vi "Service Mode Test Data.vi"(5 "High\\Low End":enum16{"HE", "LE"}(ring), 9 "Switch":T1=enum."Test 1 - Fault Codes") -> (8 "Switch Message":string)   [LabVIEW 2016, in "TL27.lvlib"]
uses:
  Projects/TL27.lvlib
  type defs/Service mode Tests.ctl
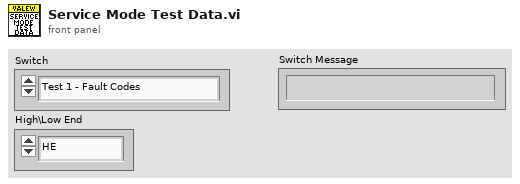
[diagram p1: front panel]
types:
  T1 = typedef "TL27.lvlib/Service mode Tests.ctl" = enum16{"Test 0 - All LEDs on", "Test 1 - Fault Codes", "Test 2 - Personality ID", "Test 3 - UI Software Ver(Crit)", "Test 4 - UI Software Ver(Non-crit)", "Test 5 - XML Ver (Non-Crit) ", "Test 6 - Hot Water Valve", "Test 7 - Cold Water Valve", "Test 8 - Fabric Softener Disp", "Test 9 - Spray Rinse Valve Check", "Test 10 - Pressure Sensor", "Test 11 - Recirc Pump", "Test 12 - Drain Pump", "Test 13 - Lid Switch", "Test 14 - Spin", "Test 15 - Agitate", "Test 16 - Clear all Fcodes", "Test 17 - Change Personality", "Test 18 - Analog Knob", "Test 19 - Bulk Dispense"}
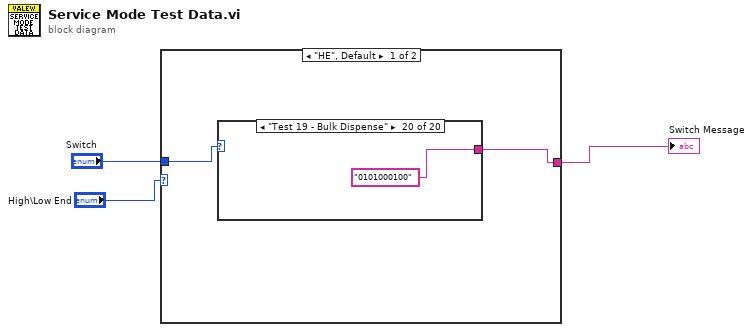
[diagram p0: block diagram]
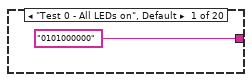
[diagram p2: hidden frame]
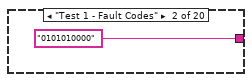
[diagram p3: hidden frame]
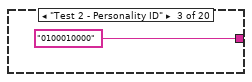
[diagram p4: hidden frame]
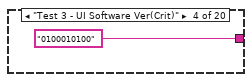
[diagram p5: hidden frame]
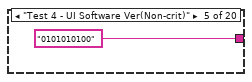
[diagram p6: hidden frame]
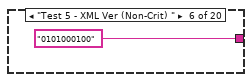
[diagram p7: hidden frame]
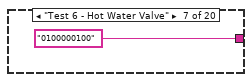
[diagram p8: hidden frame]
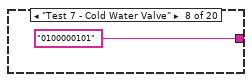
[diagram p9: hidden frame]
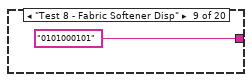
[diagram p10: hidden frame]
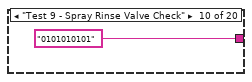
[diagram p11: hidden frame]
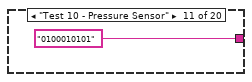
[diagram p12: hidden frame]
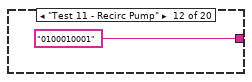
[diagram p13: hidden frame]
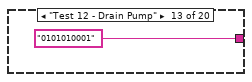
[diagram p14: hidden frame]
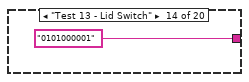
[diagram p15: hidden frame]
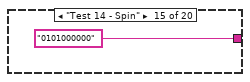
[diagram p16: hidden frame]
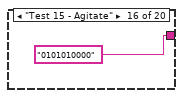
[diagram p17: hidden frame]
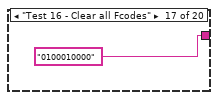
[diagram p18: hidden frame]
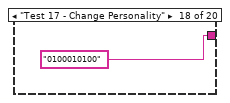
[diagram p19: hidden frame]
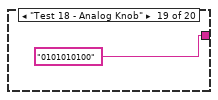
[diagram p20: hidden frame]
diagram:
  n1 = case shown="\"HE\", Default" "High\\Low End" {
    tunnel: [w4 w26] -> w3
    tunnel: "Switch" -> [w5 w27]
    frame "HE", Default {
      n2 = case shown="\"Test 19 - Bulk Dispense\"" w5 {
        tunnel: ["0101000000" ("Message") "0101010000" ("Message") "0100010000" ("Message") "0100010100" ("Message") "0101010100" ("Message") "0101000100" ("Message") "0100000100" ("Message") "0100000101" ("Message") "0101000101" ("Message") "0101010101" ("Message") "0100010101" ("Message") "0100010001" ("Message") "0101010001" ("Message") "0101000001" ("Message") "0101000000" ("Message") "0101010000" ("Message") "0100010000" ("Message") "0100010100" ("Message") "0101010100" ("Message") "0101000100" ("Message")] -> w4
        frame "Test 0 - All LEDs on", Default {
        }
        frame "Test 1 - Fault Codes" {
        }
        frame "Test 2 - Personality ID" {
        }
        frame "Test 3 - UI Software Ver(Crit)" {
        }
        frame "Test 4 - UI Software Ver(Non-crit)" {
        }
        frame "Test 5 - XML Ver (Non-Crit) " {
        }
        frame "Test 6 - Hot Water Valve" {
        }
        frame "Test 7 - Cold Water Valve" {
        }
        frame "Test 8 - Fabric Softener Disp" {
        }
        frame "Test 9 - Spray Rinse Valve Check" {
        }
        frame "Test 10 - Pressure Sensor" {
        }
        frame "Test 11 - Recirc Pump" {
        }
        frame "Test 12 - Drain Pump" {
        }
        frame "Test 13 - Lid Switch" {
        }
        frame "Test 14 - Spin" {
        }
        frame "Test 15 - Agitate" {
        }
        frame "Test 16 - Clear all Fcodes" {
        }
        frame "Test 17 - Change Personality" {
        }
        frame "Test 18 - Analog Knob" {
        }
        frame "Test 19 - Bulk Dispense" {
        }
      }
    }
    frame "LE" {
      n3 = case shown="\"Test 0 - All LEDs on\", Default" w27 {
        tunnel: ["0101010000" ("Message") "0100010000" ("Message") "0100000000" ("Message") "0101000000" ("Message") "0101000100" ("Message") "0100000100" ("Message") "0100010100" ("Message") "0100010101" ("Message") "0100000101" ("Message") "0101000101" ("Message") "0101000001" ("Message") "0100000001" ("Message") "0100010001" ("Message") "0101010001" ("Message") "0101010000" ("Message") "0100010000" ("Message") "0100000000" ("Message") "0101000000" ("Message") "0101000100" ("Message") "0000000100" ("Message")] -> w26
        frame "Test 0 - All LEDs on", Default {
        }
        frame "Test 1 - Fault Codes" {
        }
        frame "Test 2 - Personality ID" {
        }
        frame "Test 3 - UI Software Ver(Crit)" {
        }
        frame "Test 4 - UI Software Ver(Non-crit)" {
        }
        frame "Test 5 - XML Ver (Non-Crit) " {
        }
        frame "Test 6 - Hot Water Valve" {
        }
        frame "Test 7 - Cold Water Valve" {
        }
        frame "Test 8 - Fabric Softener Disp" {
        }
        frame "Test 9 - Spray Rinse Valve Check" {
        }
        frame "Test 10 - Pressure Sensor" {
        }
        frame "Test 11 - Recirc Pump" {
        }
        frame "Test 12 - Drain Pump" {
        }
        frame "Test 13 - Lid Switch" {
        }
        frame "Test 14 - Spin" {
        }
        frame "Test 15 - Agitate" {
        }
        frame "Test 16 - Clear all Fcodes" {
        }
        frame "Test 17 - Change Personality" {
        }
        frame "Test 18 - Analog Knob" {
        }
        frame "Test 19 - Bulk Dispense" {
        }
      }
    }
  }
  "Switch Message" <- w3
